vi "Write enqueuer.vi"(8 "error in (no error)":errorcluster, 10 "enqueuer":string, 11 "Pack Message for Shipping  in":refnum<class "Pack Message for Shipping .lvclass">) -> (0 "error out":errorcluster, 3 "Pack Message for Shipping  out":refnum<class "Pack Message for Shipping .lvclass">)   [LabVIEW 2014, in "Controller.lvlib" / "Pack Message for Shipping .lvclass"]
uses:
  Pack Message for Shipping .lvclass
  Pack Message for Shipping .lvclass/Pack Message for Shipping .ctl
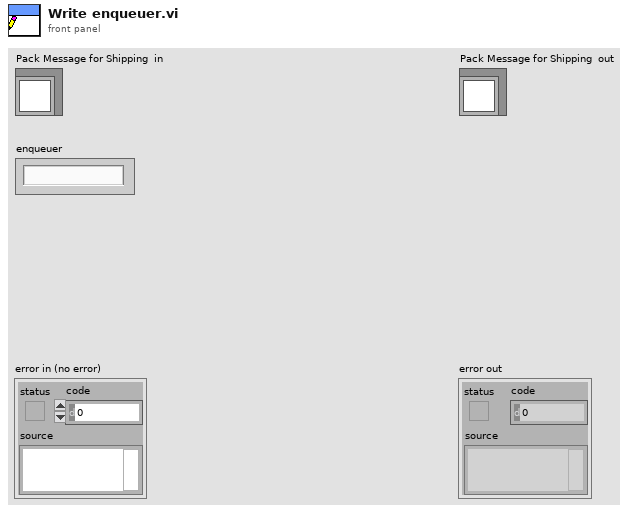
[diagram p1: front panel]
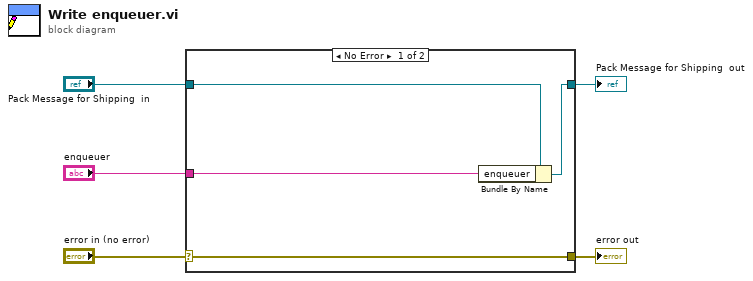
[diagram p0: block diagram]
diagram:
  n1 = case shown="No Error" "error in (no error)" {
    selector: "error in (no error)" -> [w9 w10]
    tunnel: [w9 w10] -> w4
    tunnel: [w7 w11] -> w2
    tunnel: "Pack Message for Shipping  in" -> [w8 w11]
    tunnel: "enqueuer" -> [w6 _]
    frame No Error {
      n2 = Bundle By Name(cluster=w8, "enqueuer"=w6) -> (w7:refnum<class "Pack Message for Shipping .lvclass">)
    }
    frame Error {
    }
  }
  "error out" <- w4
  "Pack Message for Shipping  out" <- w2
